vi "SetPriority.vi"(8 "error in (no error)":errorcluster, 11 "PRIORITY":enum16{"NORMAL", "IDLE", "HIGH", "REALTIME"}(ring)=enum."REALTIME") -> (0 "error out":errorcluster)   [LabVIEW 2018]
uses:
  kernel32.dll
panel:
  out "Numeric 2":u32
  out "Numeric":u32
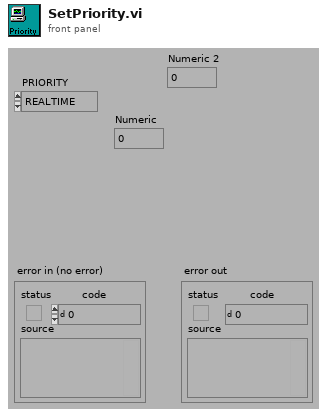
[diagram p1: front panel]
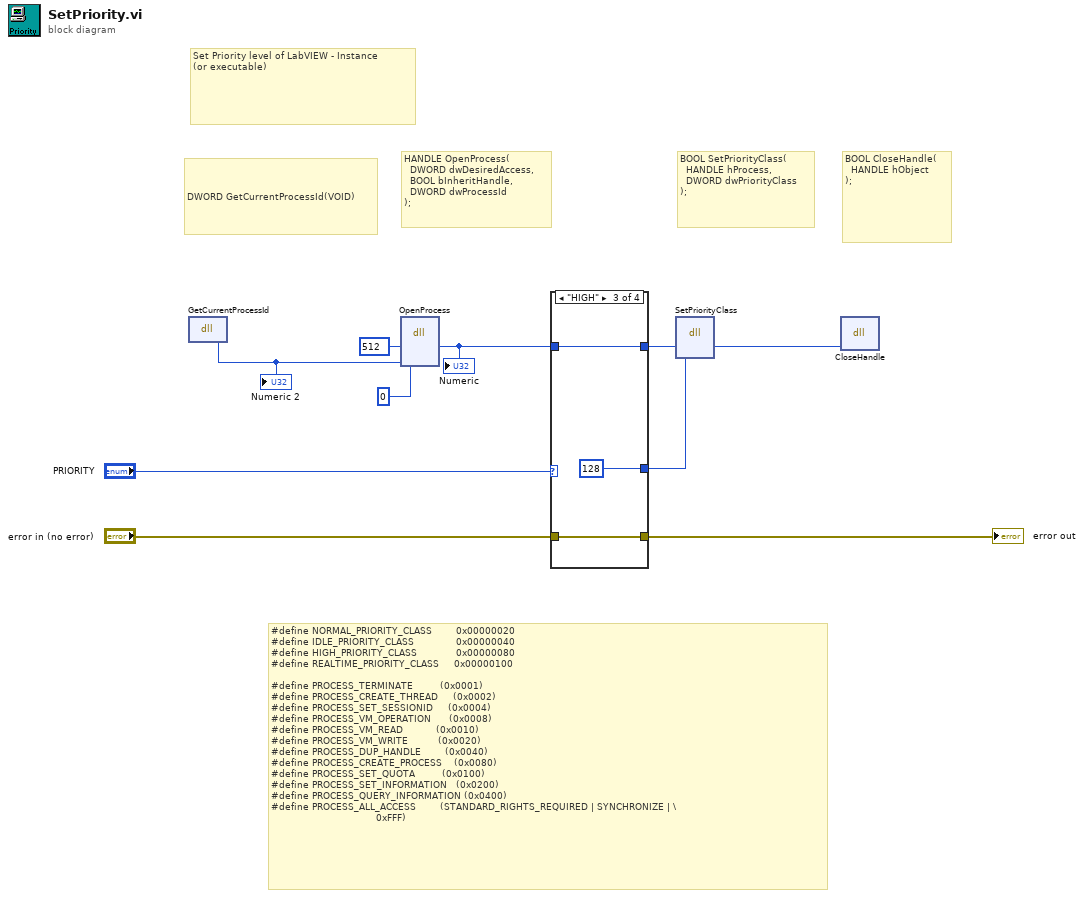
[diagram p0: block diagram]
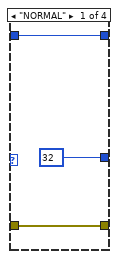
[diagram p2: hidden frame]
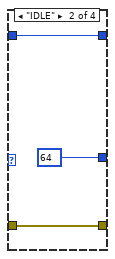
[diagram p3: hidden frame]
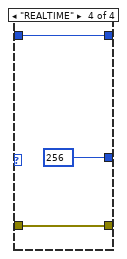
[diagram p4: hidden frame]
diagram:
  # "Set Priority level of LabVIEW - Instance \n(or executable)"
  # "BOOL SetPriorityClass(\n  HANDLE hProcess,\n  DWORD dwPriorityClass\n);"
  # "DWORD GetCurrentProcessId(VOID)"
  # "BOOL CloseHandle(\n  HANDLE hObject\n);"
  # "HANDLE OpenProcess(\n  DWORD dwDesiredAccess,\n  BOOL bInheritHandle,\n  DWORD dwProcessId\n);"
  # "#define NORMAL_PRIORITY_CLASS        0x00000020\n#define IDLE_PRIORITY_CLASS              0x00000040\n#define HIGH_PRIORITY_CLASS             0x00000080\n#define REALTIME_PRIORITY_CLASS     0x00000100\n\n#define PROCESS_TERMINATE         (0x0001)  \n#define PROCESS_CREATE_THREAD     (0x0002)  \n#define PROCESS_SET_SESSIONID     (0x0004)  \n#define PROCESS_VM_OPERATION      (0x0008)  \n#define PROCESS_VM_READ           (0x0010)  \n#define PROCESS_VM_WRITE          (0x0020)  \n#define PROCESS_DUP_HANDLE        (0x0040)  \n#define PROCESS_CREATE_PROCESS    (0x0080)  \n#define PROCESS_SET_QUOTA         (0x0100)  \n#define PROCESS_SET_INFORMATION   (0x0200)  \n#define PROCESS_QUERY_INFORMATION (0x0400)  \n#define PROCESS_ALL_ACCESS        (STANDARD_RIGHTS_REQUIRED | SYNCHRONIZE | \\\n                                   0xFFF)"
  n1 = dll-call lib="kernel32.dll" fn="GetCurrentProcessId"() -> (w8:u32)  [unwired: 3 in, 2 out]
  "Numeric 2" <- w8
  n2 = dll-call lib="kernel32.dll" fn="OpenProcess"("dwDesiredAccess"=u32 512, "bInheritHandle"=u32 0, "dwProcessID"=w8) -> (w5:u32)  [unwired: 6 in, 2 out]
  "Numeric" <- w5
  n3 = case shown="\"HIGH\"" "PRIORITY" {
    tunnel: [u32 32 u32 64 u32 128 u32 256] -> w2
    tunnel: w5 -> [w12 w15 w18 w21]
    tunnel: [w12 w15 w18 w21] -> w1
    tunnel: "error in (no error)" -> [w11 w14 w17 w20]
    tunnel: [w11 w14 w17 w20] -> w4
    frame "NORMAL" {
    }
    frame "IDLE" {
    }
    frame "HIGH" {
    }
    frame "REALTIME" {
    }
  }
  "error out" <- w4
  n4 = dll-call lib="kernel32.dll" fn="SetPriorityClass"("hProcess"=w1, "dwPriorityClass"=w2) -> ("hProcess"=w3:u32)  [unwired: 5 in, 2 out]
  n5 = dll-call lib="kernel32.dll" fn="CloseHandle"("hObject"=w3) -> ()  [unwired: 5 in, 2 out]
